vi "multi_sensor.vi"() -> ()   [LabVIEW 2012]
uses:
  <vilib>/Instr/_visa.llb/VISA Configure Serial Port (Instr).vi
panel:
  out "power":dbl(slide) scale=0.0..200.0
  out "1":u32
  out "read buffer 2":string
  out "2":u32
  in  "Blank Button":bool
  out "read buffer":string
  out "time string":string
  out "date string":string
  out "Temprature Value":dbl
  out "Heart Rate":dbl
  out "Temprature":dbl(slide) scale=0.0..100.0
  out "?":dbl(knob) scale=0.0..140.0
  in  "File Path Control":path
  in  "VISA resource name":refnum<visa-resource-name>
  in  "Stop Button":bool
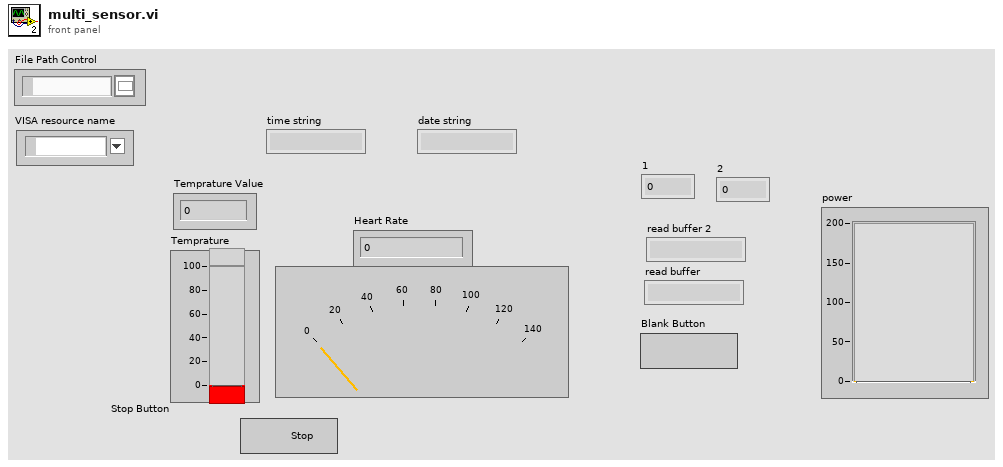
[diagram p1: front panel]
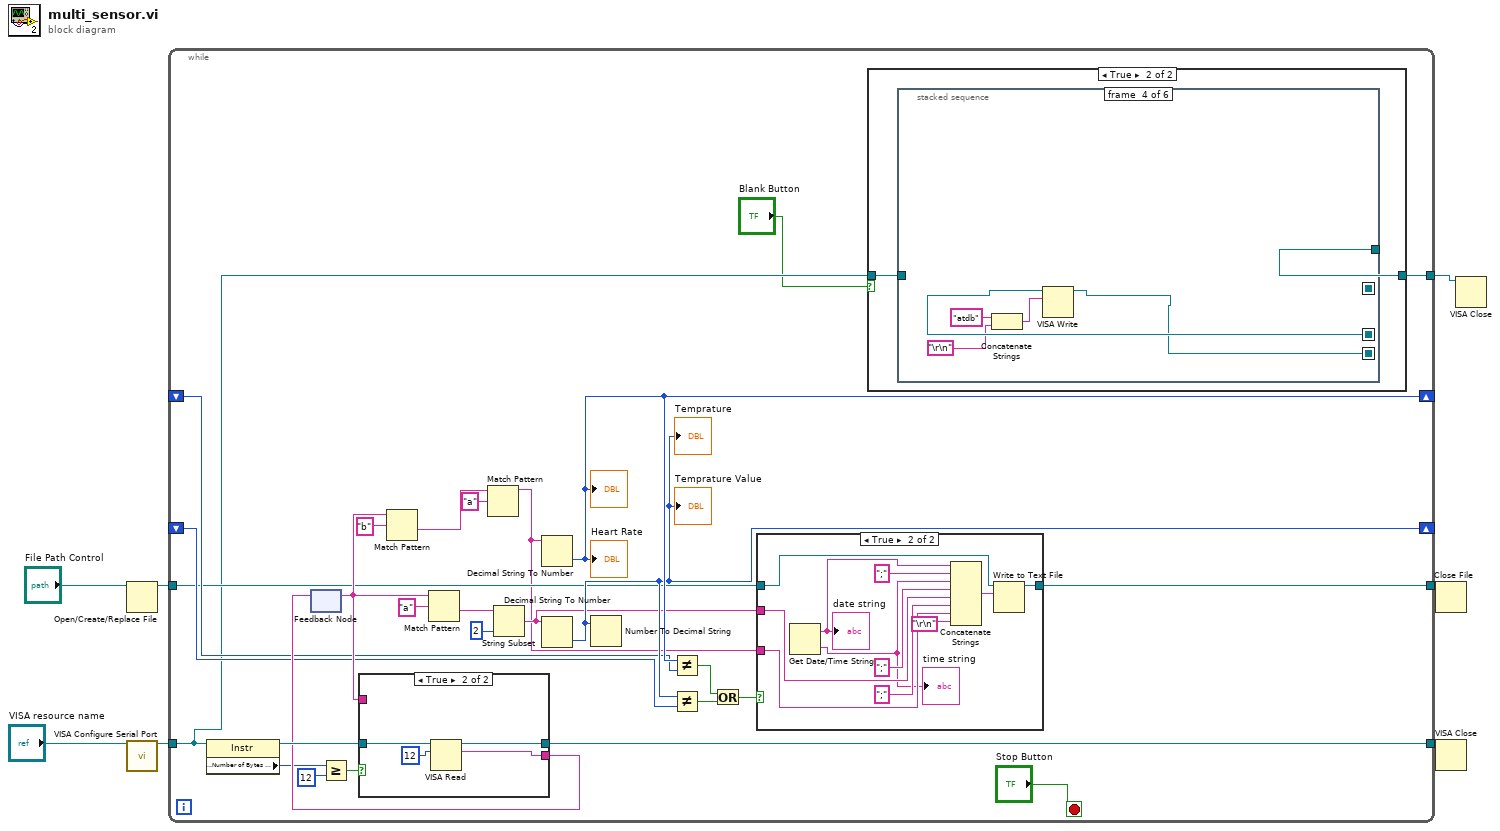
[diagram p0: block diagram]
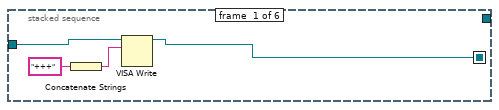
[diagram p3: hidden frame]
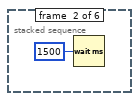
[diagram p4: hidden frame]
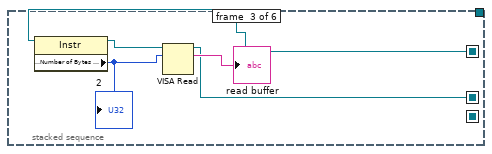
[diagram p5: hidden frame]
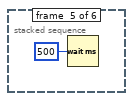
[diagram p6: hidden frame]
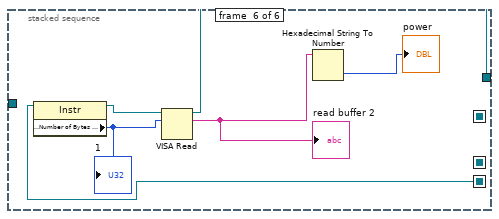
[diagram p7: hidden frame]
diagram:
  n1 = Open/Create/Replace File(file path (use dialog)="File Path Control") -> (refnum out=w4:refnum<file>)  [unwired: 5 in, 2 out]
  n2 = call-poly "VISA Configure Serial Port"("VISA resource name"="VISA resource name") -> ("VISA resource name out"=w7:refnum<visa-resource-name>)  [unwired: 13 in, 1 out]
  n3 = while {
    tunnel: w7 -> [w10]
    tunnel: [w25] -> w6
    tunnel: w4 -> [w16]
    tunnel: [w17] -> w3
    shift-right: [w21] -> _
    shift-left: _ -> [w19]
    shift-right: [w20] -> _
    shift-left: _ -> [w18]
    tunnel: [w9] -> w1
    stop <- "Stop Button" stop-if-true
    n4 = property class="Instr"(reference=w10) -> (reference out=w31:refnum<visa-resource-name>, "Serial Settings:Number of Bytes at Serial Port"=w28:u32)  [unwired: 1 in, 1 out]
    n5 = feedback #1() -> (w29:string)  [unwired: 1 in]
    n6 = Greater Or Equal?(x=w28, y=u32 12) -> (x >= y?=w26:bool)
    n7 = case shown="True" w26 {
      tunnel: [w73 w78] -> w30
      tunnel: w31 -> [w74 w77]
      tunnel: [w74 w76] -> w25
      tunnel: w29 -> [w73 _]
      frame False {
      }
      frame True {
        n8 = VISA Read(VISA resource name=w77, byte count=u32 12) -> (VISA resource name out=w76:refnum<visa-resource-name>, read buffer=w78:string)  [unwired: 1 in, 2 out]
      }
    }
    n9 = feedback-in #1(w30) -> ()
    n10 = Match Pattern(string=w29, regular expression="b") -> (after substring=w13:string)  [unwired: 1 in, 3 out]
    n11 = Match Pattern(string=w29, regular expression="a") -> (after substring=w15:string)  [unwired: 1 in, 3 out]
    n12 = Match Pattern(string=w13, regular expression="a") -> (before substring=w11:string)  [unwired: 1 in, 3 out]
    n13 = String Subset(string=w15, length (rest)=2 ("length (rest)")) -> (substring=w14:string)  [unwired: 1 in]
    n14 = Decimal String To Number(string=w11) -> (number=w21:i32)  [unwired: 2 in, 1 out]
    "?" <- w21
    "Heart Rate" <- w21
    n15 = Decimal String To Number(string=w14) -> (number=w20:i32)  [unwired: 2 in, 1 out]
    "Temprature" <- w20
    "Temprature Value" <- w20
    n16 = Number To Decimal String(number=w20) -> ()  [unwired: 1 in, 1 out]
    n17 = Not Equal?(x=w21, y=w19) -> (x != y?=w24:bool)
    n18 = Not Equal?(x=w20, y=w18) -> (x != y?=w23:bool)
    n19 = Or(x=w24, y=w23) -> (x .or. y?=w22:bool)
    n20 = case shown="True" w22 {
      tunnel: [w61 w72] -> w17
      tunnel: w16 -> [w61 w71]
      tunnel: w14 -> [_ w67]
      tunnel: w11 -> [_ w65]
      frame False {
      }
      frame True {
        n21 = Get Date/Time String() -> (date string=w70:string, time string=w62:string)  [unwired: 3 in]
        "date string" <- w70
        "time string" <- w62
        n22 = Concatenate Strings(w70, ";" ("string"), w62, ";" ("string"), w67, ";" ("string"), w65, "\r\n") -> (w64:string)
        n23 = Write to Text File(file (use dialog)=w71, text=w64) -> (refnum out=w72:refnum<file>)  [unwired: 2 in, 2 out]
      }
    }
    n24 = case shown="True" "Blank Button" {
      tunnel: w10 -> [w36 w38]
      tunnel: [w36 w37] -> w9
      frame False {
      }
      frame True {
        n25 = stacked-sequence {
          seq-local: [w39 _ _ _ _ _] -> [_ _ w46 _ _ _]
          seq-local: [_ _ w44 _ _ _] -> [_ _ _ w51 _ _]
          seq-local: [_ _ _ w49 _ _] -> [_ _ _ _ _ w58]
          tunnel: w38 -> [w42 _ _ _ _ _]
          tunnel: [_ _ _ _ _ w57] -> w37
          frame #0 {
            n26 = Concatenate Strings("+++" ("string")) -> (w40:string)
            n27 = VISA Write(VISA resource name=w42, write buffer=w40) -> (VISA resource name out=w39:refnum<visa-resource-name>)  [unwired: 1 in, 2 out]
          }
          frame #1 {
            n28 = Wait (ms)(milliseconds to wait=u32 1500) -> ()  [unwired: 1 out]
          }
          frame #2 {
            n29 = property class="Instr"(reference=w46) -> (reference out=w45:refnum<visa-resource-name>, "Serial Settings:Number of Bytes at Serial Port"=w48:u32)  [unwired: 1 in, 1 out]
            "2" <- w48
            n30 = VISA Read(VISA resource name=w45, byte count=w48) -> (VISA resource name out=w44:refnum<visa-resource-name>, read buffer=→"read buffer":string)  [unwired: 1 in, 2 out]
          }
          frame #3 {
            n31 = Concatenate Strings("atdb" ("string"), "\r\n") -> (w52:string)
            n32 = VISA Write(VISA resource name=w51, write buffer=w52) -> (VISA resource name out=w49:refnum<visa-resource-name>)  [unwired: 1 in, 2 out]
          }
          frame #4 {
            n33 = Wait (ms)(milliseconds to wait=u32 500) -> ()  [unwired: 1 out]
          }
          frame #5 {
            n34 = property class="Instr"(reference=w58) -> (reference out=w59:refnum<visa-resource-name>, "Serial Settings:Number of Bytes at Serial Port"=w60:u32)  [unwired: 1 in, 1 out]
            "1" <- w60
            n35 = VISA Read(VISA resource name=w59, byte count=w60) -> (VISA resource name out=w57:refnum<visa-resource-name>, read buffer=w56:string)  [unwired: 1 in, 2 out]
            "read buffer 2" <- w56
            n36 = Hexadecimal String To Number(string=w56) -> (number=→"power":u32)  [unwired: 2 in, 1 out]
          }
        }
      }
    }
  }
  n37 = Close File(refnum=w3) -> ()  [unwired: 1 in, 2 out]
  n38 = VISA Close(VISA resource name=w6) -> ()  [unwired: 1 in, 1 out]
  n39 = VISA Close(VISA resource name=w1) -> ()  [unwired: 1 in, 1 out]
